vi "check if done.vi"(8 "error in (no error)":errorcluster, 11 "Autofocus in":refnum<class "Autofocus.lvclass">) -> (0 "error out":errorcluster, 3 "Autofocus out":refnum<class "Autofocus.lvclass">)   [LabVIEW 2012, in "Autofocus.lvclass"]
uses:
  Autofocus.lvclass
  Autofocus.lvclass/Autofocus.ctl
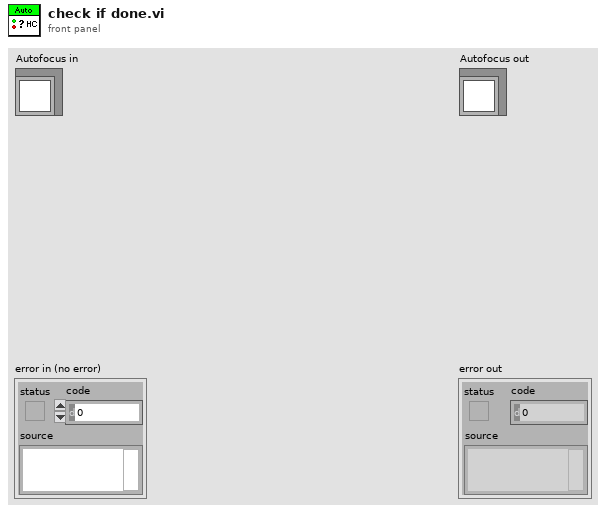
[diagram p1: front panel]
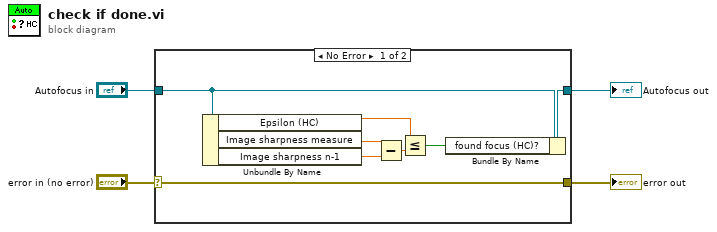
[diagram p0: block diagram]
diagram:
  n1 = case shown="No Error" "error in (no error)" {
    selector: "error in (no error)" -> [w12 w14]
    tunnel: [w12 w14] -> w3
    tunnel: [w5 w13] -> w1
    tunnel: "Autofocus in" -> [w7 w13]
    frame No Error {
      n2 = Unbundle By Name(w7) -> ("Epsilon (HC)"=w8:dbl, "Image sharpness measure"=w11:dbl, "Image sharpness n-1"=w10:dbl)
      n3 = Subtract(x=w11, y=w10) -> (x-y=w9:dbl)
      n4 = Less Or Equal?(x=w8, y=w9) -> (x <= y?=w6:bool)
      n5 = Bundle By Name(cluster=w7, "found focus (HC)?"=w6) -> (w5:refnum<class "Autofocus.lvclass">)
    }
    frame Error {
    }
  }
  "error out" <- w3
  "Autofocus out" <- w1
